vi "Remove Variable Source File in Map.vi"(7 "String":string, 8 "error in (no error)":errorcluster, 9 "dup path":path, 10 "Content":string, 11 "Variable-FileMap":variant) -> (0 "error out":errorcluster, 1 "No Source Any More?":bool, 3 "Variant":variant)   [LabVIEW 2017, in "INI-Static-Variable-Support.lvlib" / "CSM-Static-Variable-Manager.lvclass"]
uses:
  CSM-Static-Variable-Manager.lvclass
  <userlib>/_NEVSTOP/Communicable State Machine(CSM)/addons/API-String-Arugments-Support/API String Arguments Support.lvlib
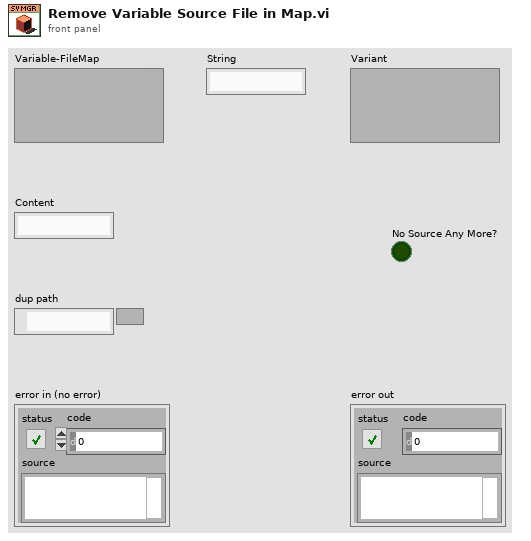
[diagram p1: front panel]
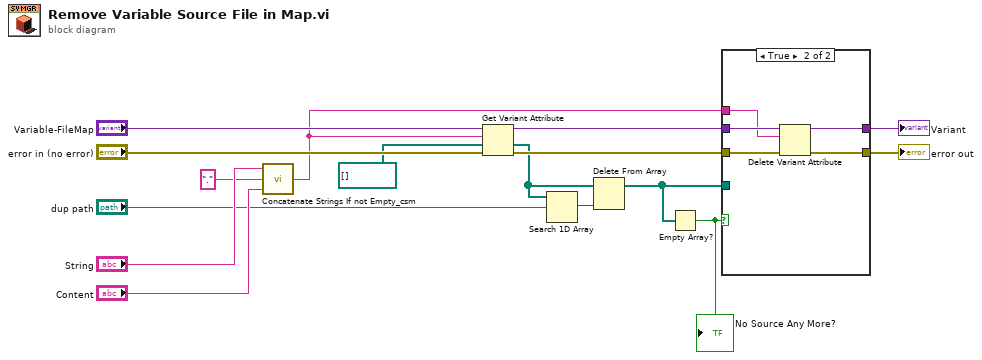
[diagram p0: block diagram]
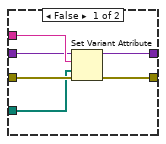
[diagram p2: hidden frame]
diagram:
  n1 = call <userlib>:"Concatenate Strings If not Empty_csm.vi"("String"="Content", "seperator(:)"=".", "prefix"="String") -> ("result"=w11:string)  [unwired: 2 in]
  n2 = Get Variant Attribute(Variant="Variable-FileMap", name=w11, default value (empty Variant)=path[] [], error in="error in (no error)") -> (duplicate Variant=w10:variant, value=w3:path[], error out=w12:errorcluster)  [unwired: 1 out]
  n3 = Search 1D Array(1D array=w3, element="dup path") -> (index of element=w4:i32)  [unwired: 1 in]
  n4 = Delete From Array(array=w3, index=w4) -> (array with subset deleted=w2:path[])  [unwired: 1 in, 1 out]
  n5 = Empty Array?(array=w2) -> (empty?=w1:bool)
  "No Source Any More?" <- w1
  n6 = case shown="True" w1 {
    tunnel: [w22 w24] -> w16
    tunnel: [w21 w26] -> w14
    tunnel: w12 -> [w20 w25]
    tunnel: w11 -> [w19 w23]
    tunnel: w10 -> [w18 w27]
    tunnel: w2 -> [w17 _]
    frame False {
      n7 = Set Variant Attribute(Variant=w18, name=w19, value=w17, error in=w20) -> (Variant out=w21:variant, error out=w22:errorcluster)  [unwired: 1 out]
    }
    frame True {
      n8 = Delete Variant Attribute(4:w25, 6:w23, 7:w27) -> (0:w24:errorcluster, 3:w26:variant)  [unwired: 1 out]
    }
  }
  "error out" <- w16
  "Variant" <- w14
